vi "LVPortGetPropertyUpdateStatusDictionary.vi"(11 "pID":string) -> (3 "Refnum out":T1)   [LabVIEW 2017]
uses:
  <userlib>/_OpenG.lib/dictionary/dictionary.llb/Dictionary Object RefNum__ogtk.ctl
  <userlib>/_OpenG.lib/dictionary/dictionary.llb/Dictionary Object RefNum - Enum__ogtk.ctl
  LVPortControlBindingGlobals.vi
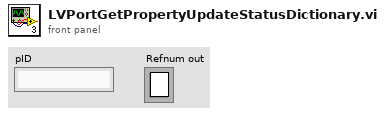
[diagram p1: front panel]
types:
  T1 = typedef "Dictionary Object RefNum__ogtk.ctl" = refnum<k1>
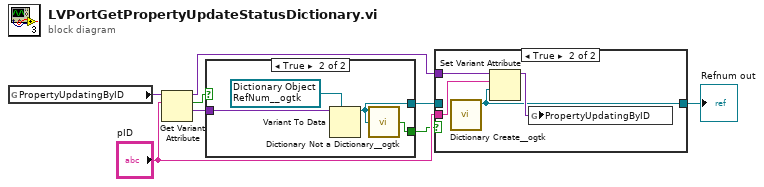
[diagram p0: block diagram]
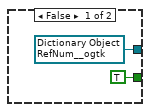
[diagram p3: hidden frame]
diagram:
  n1 = global read "LVPortControlBindingGlobals.vi" "PropertyUpdatingByID"() -> (w6:variant)
  n2 = Get Variant Attribute(Variant=w6, name="pID") -> (duplicate Variant=w1:variant, found=w2:bool, value=w3:variant)  [unwired: 2 in, 1 out]
  n3 = case shown="True" w2 {
    tunnel: w3 -> [_ w13]
    tunnel: [TRUE w11] -> w4
    tunnel: [w9 w12] -> w5
    frame False {
      w9 = T1 refnum items=["Dictionary"] ("dictionary out")
    }
    frame True {
      w14 = T1 refnum items=["Dictionary"] ("dictionary out")
      n4 = Variant To Data(type=w14, Variant=w13) -> (data=w12:T1)  [unwired: 1 in, 1 out]
      n5 = call <userlib>:"Dictionary Not a Dictionary__ogtk.vi"("dictionary"=w12) -> ("not a dictionary?"=w11:bool)
    }
  }
  n6 = case shown="True" w4 {
    tunnel: w5 -> [w15 _]
    tunnel: w1 -> [_ w19]
    tunnel: "pID" -> [_ w17]
    tunnel: [w15 w16] -> w8
    frame False {
    }
    frame True {
      n7 = call <userlib>:"Dictionary Create__ogtk.vi"() -> ("dictionary out"=w16:T1)  [unwired: 10 in, 1 out]
      n8 = Set Variant Attribute(Variant=w19, name=w17, value=w16) -> (Variant out=w18:variant)  [unwired: 1 in, 2 out]
      n9 = global write "LVPortControlBindingGlobals.vi" "PropertyUpdatingByID"(w18) -> ()
    }
  }
  "Refnum out" <- w8
